vi "api_vi_tree.vi"() -> ()   [LabVIEW 2020, in "graph.lvlib"]
uses:
  graph.lvlib
  api/DiGraph/DiGraph.lvclass
  api/Graph/Graph.lvclass
  api/Edge/Edge.lvclass
  api/Node/Node.lvclass
panel:
  out "new edge":refnum<class "Edge.lvclass">
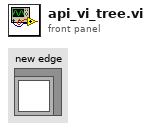
[diagram p1: front panel]
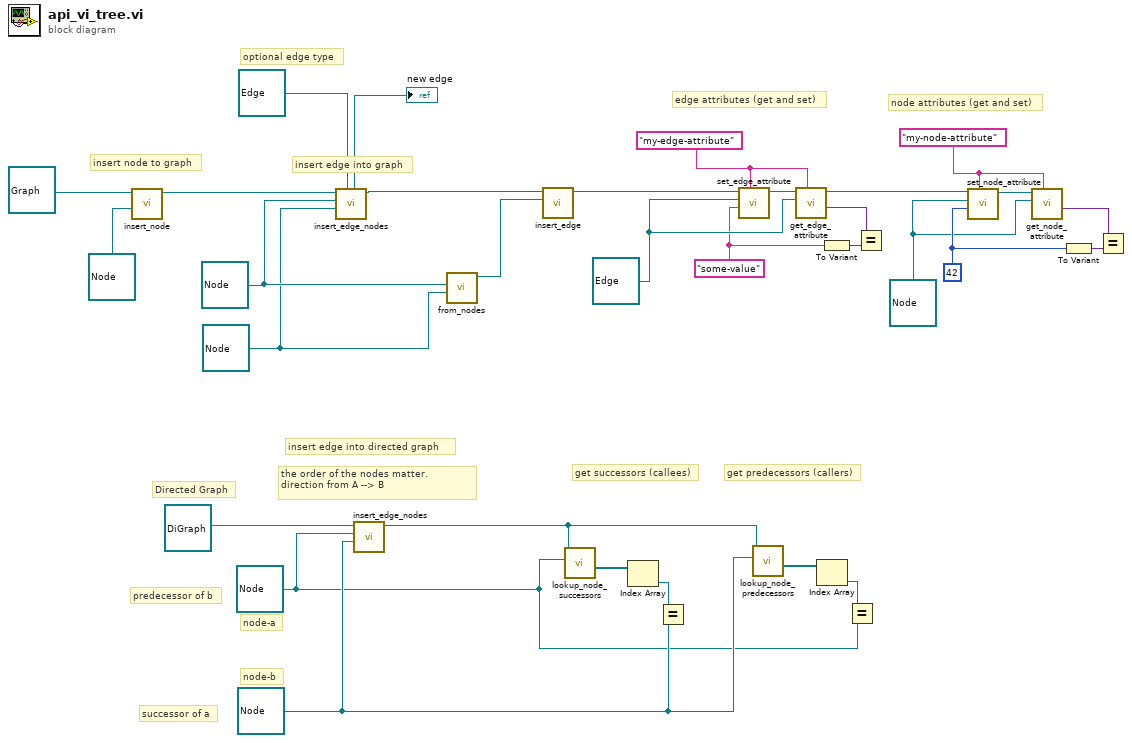
[diagram p0: block diagram]
diagram:
  w10 = 42 ("attribute-name")
  w9 = refnum<class "Node.lvclass"> refnum ("Graph.lvlib:Node.lvclass")
  w13 = "my-node-attribute" ("attribute-name")
  w19 = refnum<class "Edge.lvclass"> refnum ("graph-lv.lvlib:Edge.lvclass")
  w17 = "some-value" ("attribute-name")
  w21 = "my-edge-attribute" ("attribute-name")
  w7 = refnum<class "Node.lvclass"> refnum ("Graph.lvlib:Node.lvclass")
  w2 = refnum<class "Node.lvclass"> refnum ("Graph.lvlib:Node.lvclass")
  w26 = refnum<class "Node.lvclass"> refnum ("Graph.lvlib:Node.lvclass")
  w27 = refnum<class "Node.lvclass"> refnum ("Graph.lvlib:Node.lvclass")
  # "insert edge into directed graph"
  # "insert edge into graph"
  # "insert node to graph"
  # "get predecessors (callers)"
  # "get successors (callees)"
  # "node attributes (get and set)"
  # "edge attributes (get and set)"
  # "the order of the nodes matter.\ndirection from A --> B"
  # "optional edge type"
  # "predecessor of b"
  # "successor of a"
  # "node-b"
  # "node-a"
  # "Directed Graph"
  n1 = call "insert_node.vi"("node"=refnum<class "Node.lvclass"> refnum ("Graph.lvlib:Node.lvclass"), "graph"=refnum<class "Graph.lvclass"> refnum ("graph.lvlib:Graph.lvclass")) -> ("graph out"=w29:refnum<class "Graph.lvclass">)  [unwired: 6 in, 3 out]
  n2 = call-dynamic "insert_edge_nodes.vi"("edge type"=refnum<class "Edge.lvclass"> refnum ("graph-lv.lvlib:Edge.lvclass"), "node-b"=w26, "node-a"=w27, "graph"=w29) -> ("graph out"=w28:refnum<class "Graph.lvclass">, "new edge"=→"new edge":refnum<class "Edge.lvclass">)  [unwired: 4 in, 2 out]
  n3 = call-dynamic "insert_edge_nodes.vi"("node-b"=w7, "node-a"=w2, "graph"=refnum<class "DiGraph.lvclass"> refnum ("Graph.lvlib:DiGraph.lvclass")) -> ("graph out"=w8:refnum<class "DiGraph.lvclass">)  [unwired: 5 in, 3 out]
  n4 = call-dynamic "from_nodes.vi"("node-b"=w26, "node-a"=w27) -> ("new edge"=w20:refnum<class "Edge.lvclass">)  [unwired: 9 in]
  n5 = call-dynamic "insert_edge.vi"("edge"=w20, "digraph"=w28) -> ("digraph out"=w23:refnum<class "Graph.lvclass">)  [unwired: 7 in, 2 out]
  n6 = call-dynamic "lookup_node_successors.vi"("node"=w2, "digraph"=w8) -> ("successors"=w6:refnum<class "Node.lvclass">[])  [unwired: 8 in, 1 out]
  n7 = Index Array(array=w6) -> (element=w5:refnum<class "Node.lvclass">)  [unwired: 1 in]
  n8 = Equal?(x=w5, y=w7) -> ()  [unwired: 1 out]
  n9 = call-dynamic "set_edge_attribute.vi"("attribute-name"=w21, "attribute-value"=w17, "edge"=w19, "graph"=w23) -> ("graph-out"=w22:refnum<class "Graph.lvclass">)  [unwired: 6 in, 1 out]
  n10 = call-dynamic "lookup_node_predecessors.vi"("node"=w7, "digraph"=w8) -> ("predecessors"=w3:refnum<class "Node.lvclass">[])  [unwired: 8 in, 1 out]
  n11 = call-dynamic "get_edge_attribute.vi"("attribute-name"=w21, "edge"=w19, "graph"=w22) -> ("attribute-value"=w18:variant, "graph-out"=w14:refnum<class "Graph.lvclass">)  [unwired: 5 in, 2 out]
  n12 = Index Array(array=w3) -> (element=w4:refnum<class "Node.lvclass">)  [unwired: 1 in]
  n13 = To Variant(anything=w17) -> (Variant=w16:variant)
  n14 = Equal?(x=w4, y=w2) -> ()  [unwired: 1 out]
  n15 = Equal?(x=w18, y=w16) -> ()  [unwired: 1 out]
  n16 = call-dynamic "set_node_attribute.vi"("attribute-name"=w13, "attribute-value"=w10, "node"=w9, "graph"=w14) -> ("graph-out"=w15:refnum<class "Graph.lvclass">)  [unwired: 6 in, 1 out]
  n17 = call-dynamic "get_node_attribute.vi"("attribute-name"=w13, "node"=w9, "graph"=w15) -> ("attribute-value"=w11:variant)  [unwired: 5 in, 3 out]
  n18 = To Variant(anything=w10) -> (Variant=w12:variant)
  n19 = Equal?(x=w11, y=w12) -> ()  [unwired: 1 out]
